vi "_complex_Mean.vi"(1 "Zin":cdb[](array[numeric])) -> (0 "Numeric":cdb)   [LabVIEW 2013]
uses:
  <vilib>/Analysis/baseanly.llb/Mean (DBL).vi
  <vilib>/Analysis/NI_AALBase.lvlib
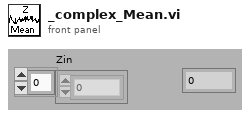
[diagram p1: front panel]
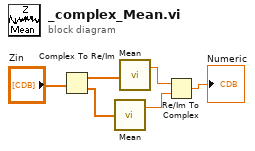
[diagram p0: block diagram]
diagram:
  n1 = Complex To Re/Im(x + iy="Zin") -> (x=w5:dbl[], y=w4:dbl[])
  n2 = call-poly <vilib>:"Mean.vi"("X"=w4) -> ("mean"=w2:dbl)  [unwired: 1 out]
  n3 = call-poly <vilib>:"Mean.vi"("X"=w5) -> ("mean"=w3:dbl)  [unwired: 1 out]
  n4 = Re/Im To Complex(1:w2, 2:w3) -> (0:→"Numeric":cdb)
